vi "in_2d_neighbor matrix.vi"(0 "array":dbl[][](array[numeric]), 5 "row index":i32, 7 "row length":i32, 9 "col index":i32, 11 "col length":i32) -> (4 "subarray":dbl[][](array[numeric]))   [LabVIEW 2010, in "NI_Gmath.lvlib"]
uses:
  NI_Gmath.lvlib
panel:
  in  "outside region":enum16{"zero", "nearest element"}(ring)
  # "2d array subset with padding"
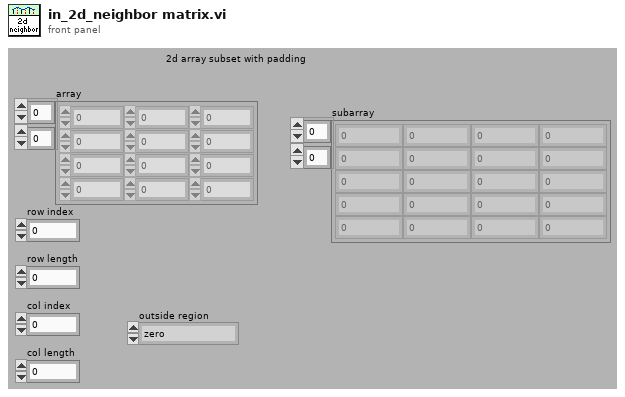
[diagram p1: front panel]
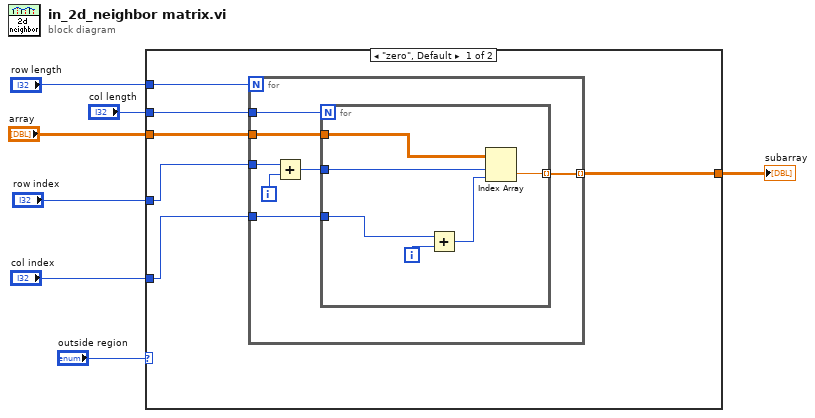
[diagram p0: block diagram]
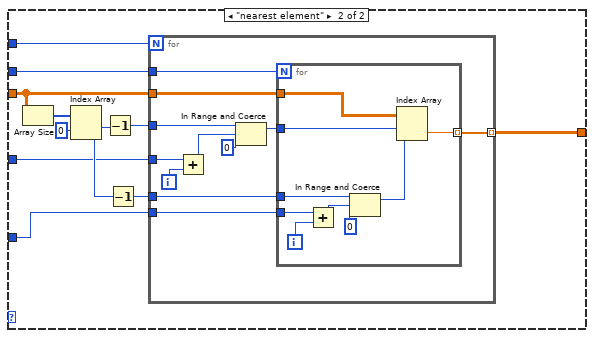
[diagram p2: hidden frame]
diagram:
  n1 = case shown="\"zero\", Default" "outside region" {
    tunnel: "row index" -> [w13 w30]
    tunnel: "col index" -> [w12 w38]
    tunnel: [w11 w37] -> w5
    tunnel: "array" -> [w10 w31]
    tunnel: "row length" -> [w9 w27]
    tunnel: "col length" -> [w8 w36]
    frame "zero", Default {
      n2 = for {
        N: w9 -> [_]
        tunnel: w8 -> [w20]
        tunnel: w13 -> [w16]
        tunnel: w12 -> [w19]
        tunnel: [w18] -> w11 mode=indexing
        tunnel: w10 -> [w17]
        i -> [w15]
        n3 = Add(x=w16, y=w15) -> (x+y=w14:i32)
        n4 = for {
          N: w20 -> [_]
          tunnel: w19 -> [w23]
          tunnel: [w26] -> w18 mode=indexing
          tunnel: w17 -> [w25]
          tunnel: w14 -> [w21]
          i -> [w24]
          n5 = Add(x=w23, y=w24) -> (x+y=w22:i32)
          n6 = Index Array(array=w25, index (row)=w21, index (col)=w22) -> (element=w26:dbl)
        }
      }
    }
    frame "nearest element" {
      n7 = Array Size(array=w31) -> (size(s)=w32:i32[])
      n8 = Index Array(array=w32, index #1=0 ("index")) -> (element #1=w34:i32, element #2=w35:i32)  [unwired: 1 in]
      n9 = Decrement(x=w34) -> (x-1=w28:i32)
      n10 = Decrement(x=w35) -> (x-1=w29:i32)
      n11 = for {
        N: w27 -> [_]
        tunnel: w36 -> [w49]
        tunnel: w30 -> [w45]
        tunnel: w38 -> [w48]
        tunnel: [w47] -> w37 mode=indexing
        tunnel: w31 -> [w46]
        tunnel: w29 -> [w41]
        tunnel: w28 -> [w40]
        i -> [w39]
        n12 = Add(x=w45, y=w39) -> (x+y=w44:i32)
        n13 = In Range and Coerce(upper limit=w40, x=w44, lower limit=0) -> (coerced(x)=w43:i32)  [unwired: 1 out]
        n14 = for {
          N: w49 -> [_]
          tunnel: w48 -> [w52]
          tunnel: [w58] -> w47 mode=indexing
          tunnel: w46 -> [w57]
          tunnel: w43 -> [w55]
          tunnel: w41 -> [w50]
          i -> [w56]
          n15 = Add(x=w52, y=w56) -> (x+y=w53:i32)
          n16 = In Range and Coerce(upper limit=w50, x=w53, lower limit=0) -> (coerced(x)=w51:i32)  [unwired: 1 out]
          n17 = Index Array(array=w57, index (row)=w55, index (col)=w51) -> (element=w58:dbl)
        }
      }
    }
  }
  "subarray" <- w5
